vi "DSF.Engine.Framework.Initialize.Plugins.Sort by Priority.vi"(8 "error in (no error)":errorcluster, 10 "Plugins":refnum<class "Plugin.lvclass">[](array[class]), 11 "Framework in":refnum<class "Framework.lvclass">) -> (0 "error out":errorcluster, 2 "sorted Plugins":refnum<class "Plugin.lvclass">[](array[class]), 3 "Framework out":refnum<class "Framework.lvclass">)   [LabVIEW 2017, in "DSF.Engine.lvlib" / "Framework.lvclass"]
uses:
  Framework.lvclass
  Plugin/Plugin.lvclass
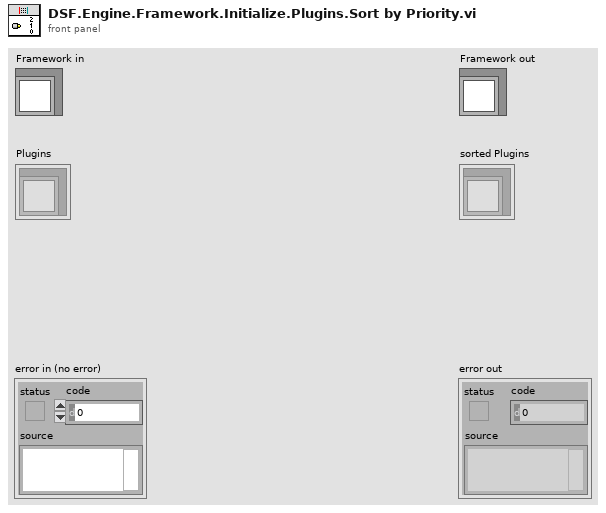
[diagram p1: front panel]
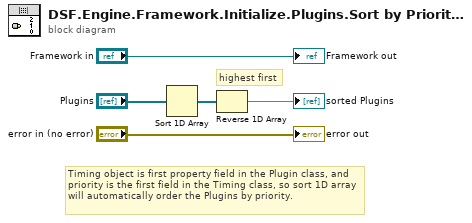
[diagram p0: block diagram]
diagram:
  # "highest first"
  # "Timing object is first property field in the Plugin class, and priority is the first field in the Timing class, so sort 1D array will automatically order the Plugins by priority."
  n1 = Sort 1D Array(array="Plugins") -> (sorted array=w4:refnum<class "Plugin.lvclass">[])
  n2 = Reverse 1D Array(array=w4) -> (reversed array=→"sorted Plugins":refnum<class "Plugin.lvclass">[])
  "error out" <- "error in (no error)"
  "Framework out" <- "Framework in"
